vi "Character_to_Dec_Num.vi"(8 "error I":errorcluster, 10 "width (-)":i16, 11 "Input Character":string) -> (0 "error O":errorcluster, 2 "Decimal String":string, 3 "Decimal Number":i32)   [LabVIEW 2011]
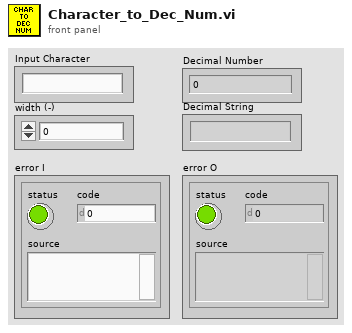
[diagram p1: front panel]
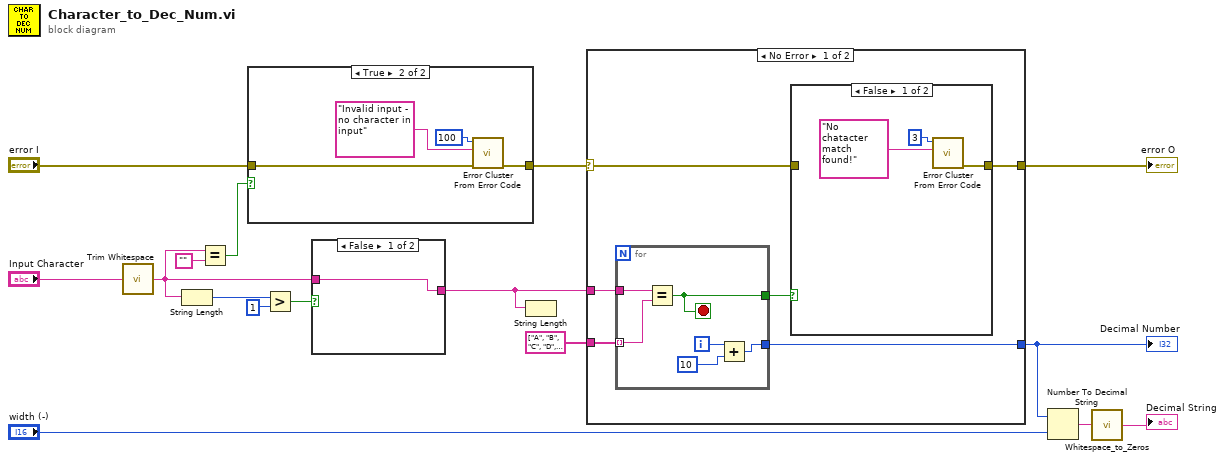
[diagram p0: block diagram]
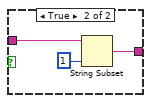
[diagram p2: hidden frame]
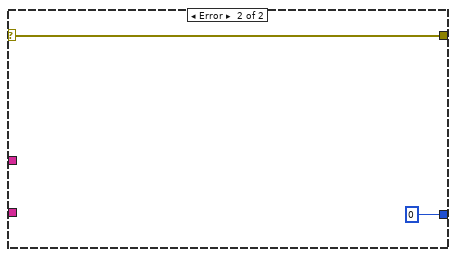
[diagram p5: hidden frame]
diagram:
  n1 = call <vilib>:"Trim Whitespace.vi"("string"="Input Character") -> ("trimmed string"=w6:string)  [unwired: 1 in]
  n2 = String Length(string=w6) -> (length=w16:i32)
  n3 = Equal?(x=w6, y="") -> (x = y?=w10:bool)
  n4 = case shown="True" w10 {
    tunnel: [w17 w18] -> w8
    tunnel: "error I" -> [w17 w21]
    frame False {
    }
    frame True {
      n5 = call <vilib>:"Error Cluster From Error Code.vi"("error in (no error)"=w21, "error message (\"\")"="Invalid input - no character in input" ("error message (\"\")"), "error code (0)"=100) -> ("error out"=w18:errorcluster)  [unwired: 6 in]
    }
  }
  n6 = Greater?(x=w16, y=1) -> (0:w7:bool)
  n7 = case shown="False" w7 {
    tunnel: w6 -> [w22 w25]
    tunnel: [w22 w23] -> w5
    frame False {
    }
    frame True {
      n8 = String Subset(string=w25, length (rest)=1 ("length (rest)")) -> (substring=w23:string)  [unwired: 1 in]
    }
  }
  n9 = String Length(string=w5) -> ()  [unwired: 1 out]
  n10 = case shown="No Error" w8 {
    selector: w8 -> [w27 w43]
    tunnel: string[] ["A", "B", "C", "D", "E", "F", "G", "H", "I", "J", "K", "L", "M", "N", "O", "P", "Q", "R", "S", "T", "U", "V", "W", "X", "Y", "Z"] -> [w31 _]
    tunnel: w5 -> [w30 _]
    tunnel: [w28 w43] -> w12
    tunnel: [w26 0] -> w4
    frame No Error {
      n11 = for {
        tunnel: w31 -> [w40] mode=indexing
        tunnel: w30 -> [w41]
        tunnel: [w39] -> w29
        tunnel: [w36] -> w26
        i -> [w38]
        stop <- w39 stop-if-true
        n12 = Equal?(x=w41, y=w40) -> (x = y?=w39:bool)
        n13 = Add(x=w38, y=10) -> (x+y=w36:i32)
      }
      n14 = case shown="False" w29 {
        tunnel: [w32 w35] -> w28
        tunnel: w27 -> [_ w35]
        frame False {
          n15 = call <vilib>:"Error Cluster From Error Code.vi"("error message (\"\")"="No chatacter match found!" ("error message (\"\")"), "error code (0)"=3) -> ("error out"=w32:errorcluster)  [unwired: 7 in]
        }
        frame True {
        }
      }
    }
    frame Error {
    }
  }
  "error O" <- w12
  "Decimal Number" <- w4
  n16 = Number To Decimal String(number=w4, width (-)="width (-)") -> (decimal integer string=w2:string)
  n17 = call "Whitespace_to_Zeros.vi"("Input String"=w2) -> ("Output String"=→"Decimal String":string)  [unwired: 6 in]
